vi "2048_game.vi"() -> ()   [LabVIEW 2021]
uses:
  gameover.ctl
  <vilib>/event_ctls.llb/eventvkey.ctl
panel:
  in  "module path 2":path
  in  "module path":path
  in  "AI":bool
  in  "player 2":bool
  in  "path 2":path
  in  "path":path
  in  "gameover 2":T1
  out "title 2":string
  out "summon_ani 2":u16[][](array[ring]) caption="Ring"
  in  "new game 2":bool
  out "P2 Score":i32
  out "Board 2":u16[][](array[ring])
  out "title":string
  in  "gameover":T1
  out "summon_ani":u16[][](array[ring]) caption="Ring"
  in  "new game":bool
  out "P1 Score":i32
  in  "stop":bool
  out "Board":u16[][](array[ring])
  # "P2控制方式\n上:W\n下:S\n左:A\n右:D"
  # "P1控制方式\n上:up\n下:down\n左:left\n右:right"
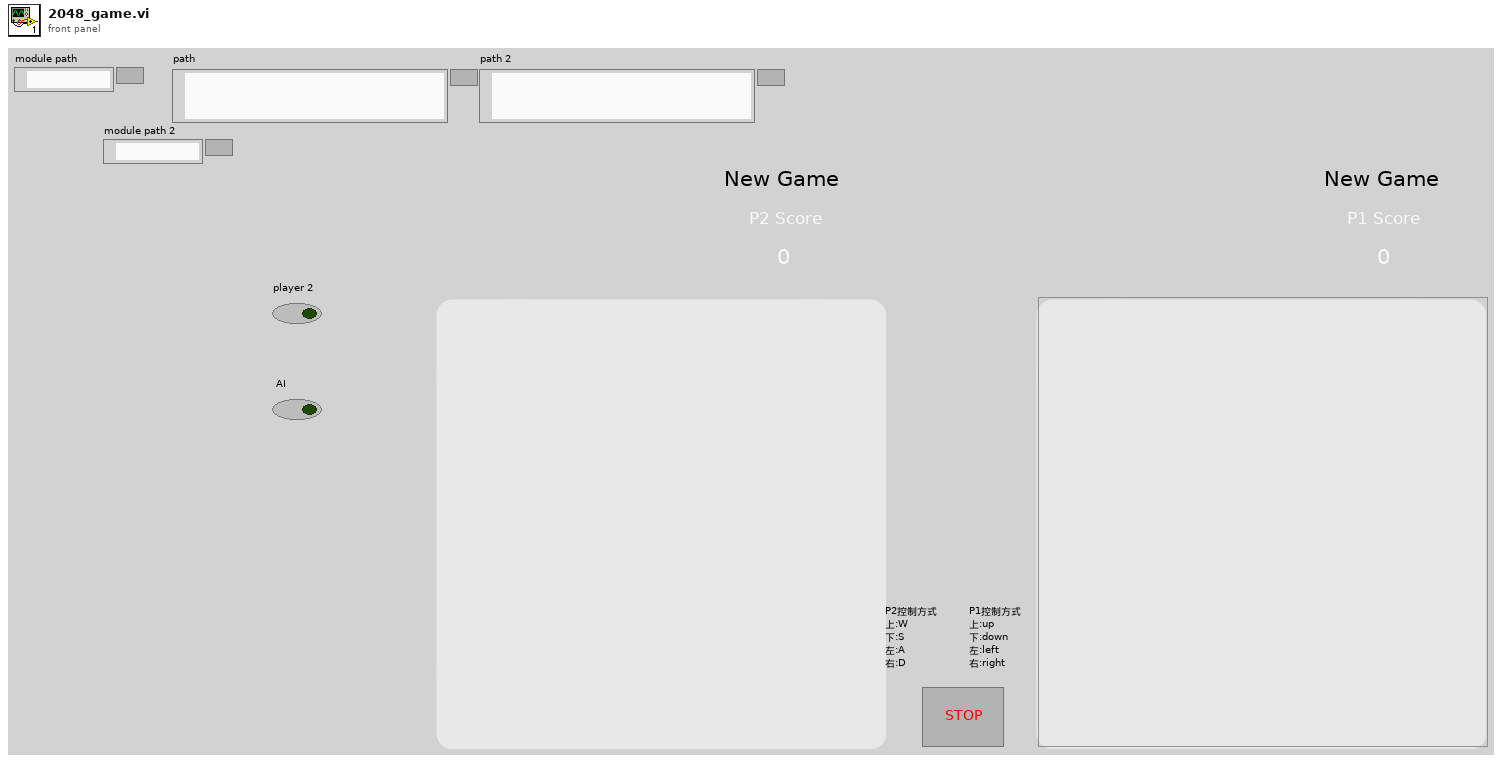
[diagram p1: front panel]
types:
  T1 = typedef "gameover.ctl" = bool
  T2 = typedef "Sound Output Task ID.ctl" = u32
  T3 = typedef "eventvkey.ctl" = enum16{"ASCII", "Enter", "Return", "Shift", "Ctrl", "Alt", "Cmd", "Opt", "Caps", "NumLock", "Clear", "Break", "Up", "Down", "Left", "Right", "Insert", "Delete", "Home", "End", "PageUp", "PageDown", "Escape", "Help", "Pause", "ScrollLock", "F1", "F2", "F3", "F4", "F5", "F6", "F7", "F8", "F9", "F10", "F11", "F12", "F13", "F14", "F15", "F16", "F17", "F18", "F19", "F20", "F21", "F22", "F23", "F24", "Play", "VolumeUp", "VolumeDown", "Mute", "Two Byte Char"}
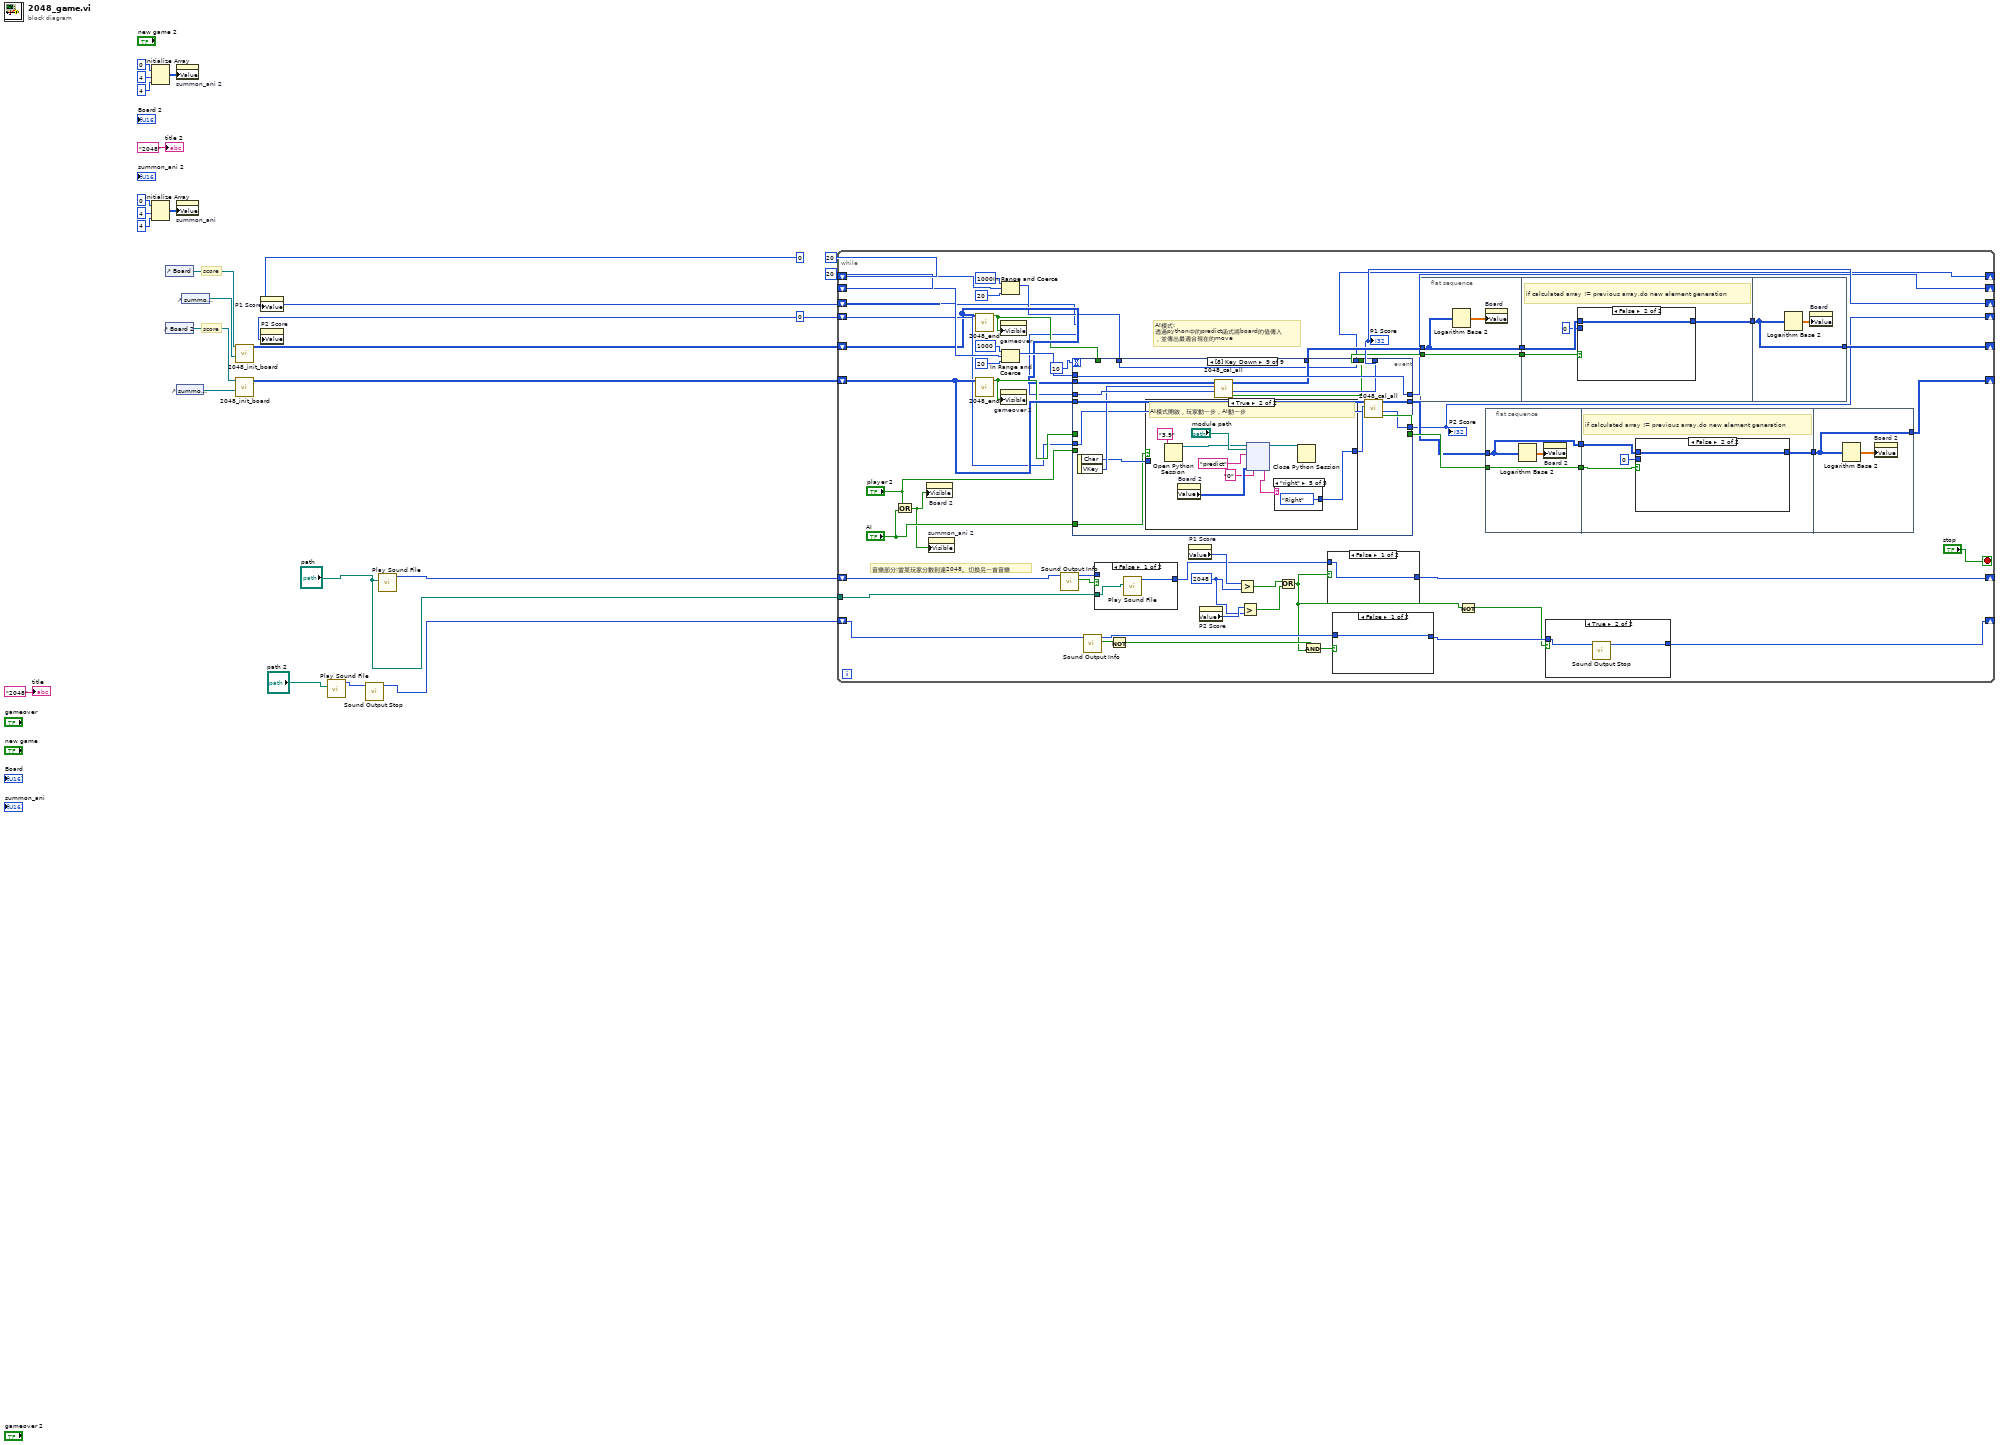
[diagram p0: block diagram]
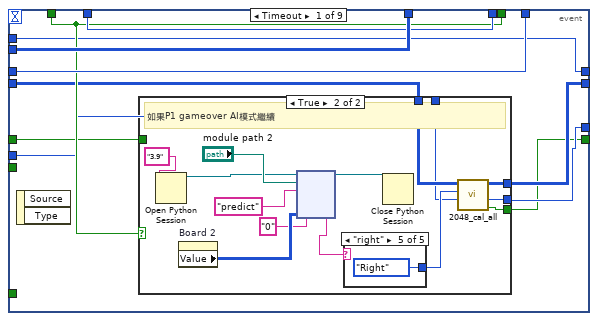
[diagram p2: hidden frame]
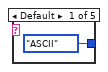
[diagram p4: hidden frame]
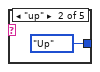
[diagram p5: hidden frame]
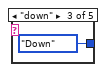
[diagram p6: hidden frame]
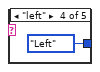
[diagram p7: hidden frame]
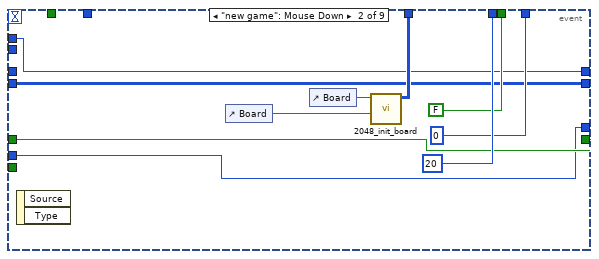
[diagram p8: hidden frame]
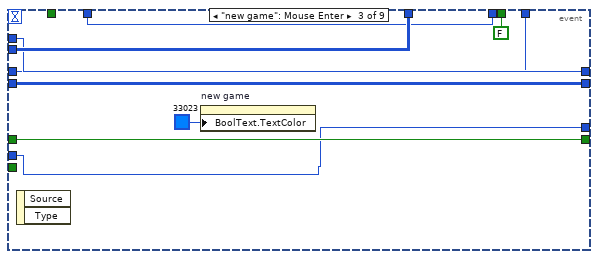
[diagram p9: hidden frame]
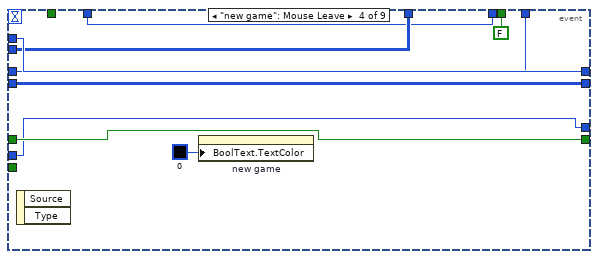
[diagram p10: hidden frame]
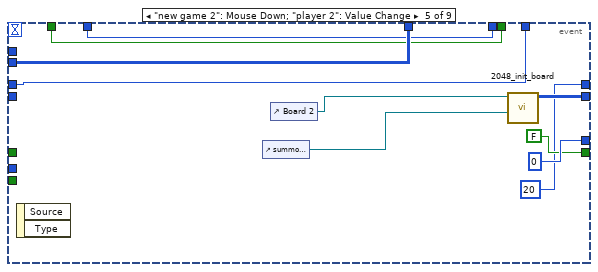
[diagram p11: hidden frame]
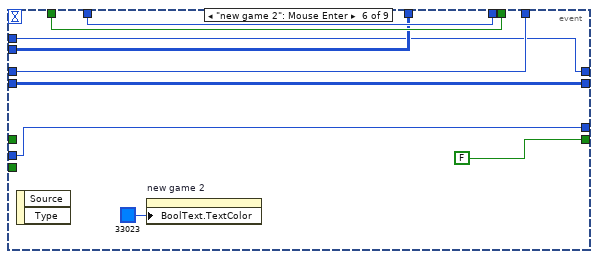
[diagram p12: hidden frame]
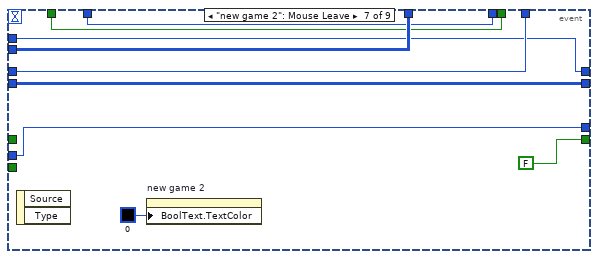
[diagram p13: hidden frame]
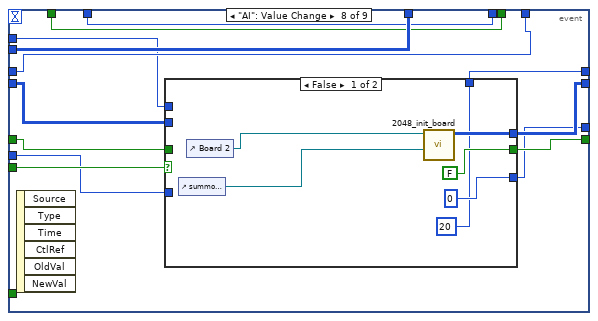
[diagram p14: hidden frame]
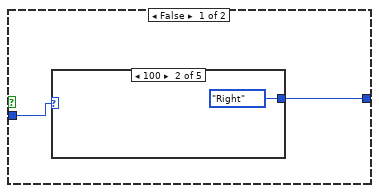
[diagram p16: hidden frame]
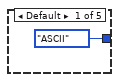
[diagram p17: hidden frame]
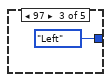
[diagram p18: hidden frame]
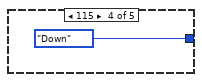
[diagram p19: hidden frame]
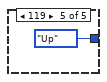
[diagram p20: hidden frame]
diagram:
  w9 = 0
  w12 = 0
  # "score"
  # "score"
  n1 = Initialize Array(0 ("element"), 4 ("dimension size"), 4 ("dimension size")) -> (w17:i32[][])
  n2 = Initialize Array(0 ("element"), 4 ("dimension size"), 4 ("dimension size")) -> (w25:i32[][])
  n3 = control-ref of="Board"() -> (w14:refnum<vi>)
  n4 = control-ref of="Board 2"() -> (w6:refnum<vi>)
  n5 = property on="summon_ani 2" class="Arr (strict)"("Value"=w17) -> ()  [unwired: 2 in, 2 out]
  n6 = property on="summon_ani" class="Arr (strict)"("Value"=w25) -> ()  [unwired: 2 in, 2 out]
  n7 = control-ref of="summon_ani 2"() -> (w7:refnum<vi>)
  n8 = control-ref of="summon_ani"() -> (w15:refnum<vi>)
  n9 = call "2048_init_board.vi"("summon_ani"=w15, "Array in"=w14) -> ("Array out"=w13:i32[][])  [unwired: 9 in]
  n10 = call "2048_init_board.vi"("summon_ani"=w7, "Array in"=w6) -> ("Array out"=w8:i32[][])  [unwired: 9 in]
  n11 = property on="P1 Score" class="DigNum (strict)"("Value"=w12) -> ()  [unwired: 2 in, 2 out]
  n12 = property on="P2 Score" class="DigNum (strict)"("Value"=w9) -> ()  [unwired: 2 in, 2 out]
  n13 = call <vilib>:"Play Sound File.vi"("path"="path 2") -> ("task ID"=w4:T2)  [unwired: 9 in, 1 out]
  n14 = call <vilib>:"Sound Output Stop.vi"("task ID"=w4) -> ("task ID out"=w3:T2)  [unwired: 9 in, 1 out]
  n15 = call <vilib>:"Play Sound File.vi"("path"="path") -> ("task ID"=w5:T2)  [unwired: 9 in, 1 out]
  n16 = while {
    shift-right: [w76] -> _
    shift-left: w13 -> [w37]
    shift-right: [w32] -> _
    shift-left: w12 -> [w34]
    shift-right: [w29] -> _
    shift-left: 20 -> [w73]
    shift-right: [w71] -> _
    shift-left: w8 -> [w44]
    shift-right: [w39] -> _
    shift-left: w9 -> [w42]
    shift-right: [w30] -> _
    shift-left: 20 -> [w72]
    shift-right: [w50] -> _
    shift-left: w5 -> [w52]
    shift-right: [w48] -> _
    shift-left: w3 -> [w51]
    tunnel: "path" -> [w53]
    stop <- "stop" stop-if-true
    w54 = 2048 ("y")
    # "AI模式: \n透過python中的predict函式將board的值傳入\n，並傳出最適合現在的move"
    # "音樂部分:當某玩家分數到達2048。切換另一首音樂"
    n17 = Or(x="player 2", y="AI") -> (x .or. y?=w27:bool)
    n18 = property on="Board 2" class="Arr (strict)"("Visible"=w27) -> ()  [unwired: 2 in, 2 out]
    n19 = property on="summon_ani 2" class="Arr (strict)"("Visible"=w27) -> ()  [unwired: 2 in, 2 out]
    n20 = call "2048_end.vi"("Array in"=w37) -> ("Boolean"=w36:bool)  [unwired: 10 in]
    n21 = call "2048_end.vi"("Array in"=w44) -> ("Boolean"=w43:bool)  [unwired: 10 in]
    n22 = property on="gameover" class="Bool (strict)"("Visible"=w36) -> ()  [unwired: 2 in, 2 out]
    n23 = property on="gameover 2" class="Bool (strict)"("Visible"=w43) -> ()  [unwired: 2 in, 2 out]
    n24 = In Range and Coerce(upper limit=1000, x=w73, lower limit=20) -> (coerced(x)=w35:i32)  [unwired: 1 out]
    n25 = In Range and Coerce(upper limit=1000, x=w72, lower limit=20) -> (coerced(x)=w38:i32)  [unwired: 1 out]
    n26 = call <vilib>:"Sound Output Info.vi"("task ID"=w52) -> ("is playing?"=w65:bool, "task ID out"=w64:T2)  [unwired: 7 in, 2 out]
    n27 = event shown="[8] Key Down" {
      selector: _ -> [_ _ _ _ _ _ _ _ _]
      dyn-events: _ -> [_ _ _ _ _ _ _ _ _]
      timeout: 10 -> [_ _ _ _ _ _ _ _ _]
      tunnel: [w86 w116 w129 w135 w151 w159 w168 w180 w206] -> w40
      tunnel: w44 -> [w87 w116 w129 w135 _ w159 w168 w175 w208]
      tunnel: [w82 w115 w130 w134 FALSE ("valid move") FALSE ("valid move") FALSE ("valid move") w178 w207] -> w41
      tunnel: [w84 w114 w124 w133 0 ("score") w153 w162 w176 w195] -> w39
      tunnel: w38 -> [w83 w117 w126 w139 _ w152 w161 w170 w205]
      tunnel: w43 -> [w81 w115 w130 w134 _ _ _ w174 _]
      tunnel: [w83 w117 w126 w139 20 w152 w161 w177 w205] -> w30
      tunnel: [w89 20 w127 w137 w146 w157 w165 w171 w197] -> w29
      tunnel: [w88 FALSE ("valid move") FALSE ("valid move") FALSE ("valid move") w144 w156 w164 w179 w198] -> w31
      tunnel: [w90 0 ("score") w125 w136 w145 w154 w163 w172 w199] -> w32
      tunnel: [w91 w118 w128 w138 w147 w155 w166 w181 w200] -> w33
      tunnel: w34 -> [w90 _ w125 w136 w145 w154 w163 w172 w203]
      tunnel: w37 -> [w91 _ w128 w138 w147 w155 w166 w181 w202]
      tunnel: w36 -> [w88 _ _ _ w144 w156 w164 w179 _]
      tunnel: w35 -> [w89 _ w127 w137 w146 w157 w165 w171 w197]
      tunnel: w42 -> [w85 w114 w124 w133 _ w153 w162 w173 w194]
      tunnel: "AI" -> [_ _ _ _ _ _ _ _ w193]
      tunnel: "player 2" -> [_ _ _ _ _ _ _ w182 _]
      event Timeout {
        n28 = event-data() -> ()  [unwired: 1 in, 2 out]
        n29 = case shown="True" w88 {
          tunnel: w87 -> [w94 w100]
          tunnel: [w94 w98] -> w86
          tunnel: w85 -> [w93 w97]
          tunnel: [w93 w96] -> w84
          tunnel: [w92 w95] -> w82
          tunnel: w81 -> [w92 _]
          frame False {
          }
          frame True {
            # "如果P1 gameover AI模式繼續"
            n30 = Open Python Session(python version="3.9" ("Python version")) -> (session out=w105:refnum<k35>)  [unwired: 2 in, 1 out]
            n31 = property on="Board 2" class="Arr (strict)"() -> ("Value"=w108:u16[][])  [unwired: 2 in, 2 out]
            n32 = node(w105, "module path 2", "predict" ("function name"), "0", w108) -> (w107:refnum<k35>, w104:string)  [unwired: 2 in, 3 out]
            n33 = case shown="\"right\"" w104 {
              tunnel: [eventvkey."ASCII" ("VKey in") eventvkey."Up" ("VKey in") eventvkey."Down" ("VKey in") eventvkey."Left" ("VKey in") eventvkey."Right" ("VKey in")] -> w99
              frame Default {
              }
              frame "up" {
              }
              frame "down" {
              }
              frame "left" {
              }
              frame "right" {
              }
            }
            n34 = Close Python Session(session in=w107) -> ()  [unwired: 1 in, 1 out]
            n35 = call "2048_cal_all.vi"("score in"=w97, "VKey in"=w99, "matrix"=w100) -> ("valid move"=w95:bool, "score out"=w96:i32, "matrix out"=w98:i32[][])  [unwired: 5 in, 1 out]
          }
        }
      }
      event "new game": Mouse Down {
        n36 = event-data() -> ()  [unwired: 1 in, 2 out]
        n37 = control-ref of="Board"() -> (w122:refnum<vi>)
        n38 = control-ref of="Board"() -> (w123:refnum<vi>)
        n39 = call "2048_init_board.vi"("summon_ani"=w122, "Array in"=w123) -> ("Array out"=w118:i32[][])  [unwired: 9 in]
      }
      event "new game": Mouse Enter {
        n40 = event-data() -> ()  [unwired: 1 in, 2 out]
        n41 = property on="new game" class="Bool (strict)"("BoolText.TextColor"=u32 33023 ("Boolean Text.Text Colors:Text Color")) -> ()  [unwired: 2 in, 2 out]
      }
      event "new game": Mouse Leave {
        n42 = event-data() -> ()  [unwired: 1 in, 2 out]
        n43 = property on="new game" class="Bool (strict)"("BoolText.TextColor"=u32 0 ("Boolean Text.Text Colors:Text Color")) -> ()  [unwired: 2 in, 2 out]
      }
      event "new game 2": Mouse Down; "player 2": Value Change {
        n44 = event-data() -> ()  [unwired: 1 in, 2 out]
        n45 = control-ref of="summon_ani 2"() -> (w143:refnum<vi>)
        n46 = control-ref of="Board 2"() -> (w142:refnum<vi>)
        n47 = call "2048_init_board.vi"("summon_ani"=w143, "Array in"=w142) -> ("Array out"=w151:i32[][])  [unwired: 9 in]
      }
      event "new game 2": Mouse Enter {
        n48 = event-data() -> ()  [unwired: 1 in, 2 out]
        n49 = property on="new game 2" class="Bool (strict)"("BoolText.TextColor"=u32 33023 ("Boolean Text.Text Colors:Text Color")) -> ()  [unwired: 2 in, 2 out]
      }
      event "new game 2": Mouse Leave {
        n50 = event-data() -> ()  [unwired: 1 in, 2 out]
        n51 = property on="new game 2" class="Bool (strict)"("BoolText.TextColor"=u32 0 ("Boolean Text.Text Colors:Text Color")) -> ()  [unwired: 2 in, 2 out]
      }
      event "AI": Value Change {
        n52 = event-data() -> ()  [unwired: 1 in, 6 out]
        n53 = case shown="False" w182 {
          tunnel: [w186 w192] -> w180
          tunnel: [0 ("score") w190] -> w176
          tunnel: [FALSE ("valid move") w191] -> w178
          tunnel: [20 w189] -> w177
          tunnel: w175 -> [_ w192]
          tunnel: w174 -> [_ w191]
          tunnel: w173 -> [_ w190]
          tunnel: w170 -> [_ w189]
          frame False {
            n54 = control-ref of="summon_ani 2"() -> (w188:refnum<vi>)
            n55 = control-ref of="Board 2"() -> (w187:refnum<vi>)
            n56 = call "2048_init_board.vi"("summon_ani"=w188, "Array in"=w187) -> ("Array out"=w186:i32[][])  [unwired: 9 in]
          }
          frame True {
          }
        }
      }
      event Key Down {
        n57 = event-data() -> ("Char"=w196:i16, "VKey"=w201:T3)  [unwired: 1 in]
        n58 = case shown="True" w193 {
          tunnel: [w210 w216] -> w204
          tunnel: w196 -> [w209 _]
          frame False {
            n59 = case shown="100" w209 {
              tunnel: [eventvkey."ASCII" ("VKey in") eventvkey."Right" ("VKey in") eventvkey."Left" ("VKey in") eventvkey."Down" ("VKey in") eventvkey."Up" ("VKey in")] -> w210
              frame Default {
              }
              frame 100 {
              }
              frame 97 {
              }
              frame 115 {
              }
              frame 119 {
              }
            }
          }
          frame True {
            # "AI模式開啟，玩家動一步，AI動一步"
            n60 = Open Python Session(python version="3.9" ("Python version")) -> (session out=w221:refnum<k35>)  [unwired: 2 in, 1 out]
            n61 = property on="Board 2" class="Arr (strict)"() -> ("Value"=w224:u16[][])  [unwired: 2 in, 2 out]
            n62 = node(w221, "module path", "predict" ("function name"), "0", w224) -> (w223:refnum<k35>, w217:string)  [unwired: 2 in, 3 out]
            n63 = case shown="\"right\"" w217 {
              tunnel: [eventvkey."ASCII" ("VKey in") eventvkey."Up" ("VKey in") eventvkey."Down" ("VKey in") eventvkey."Left" ("VKey in") eventvkey."Right" ("VKey in")] -> w216
              frame Default {
              }
              frame "up" {
              }
              frame "down" {
              }
              frame "left" {
              }
              frame "right" {
              }
            }
            n64 = Close Python Session(session in=w223) -> ()  [unwired: 1 in, 1 out]
          }
        }
        n65 = call "2048_cal_all.vi"("score in"=w203, "VKey in"=w201, "matrix"=w202) -> ("valid move"=w198:bool, "score out"=w199:i32, "matrix out"=w200:i32[][])  [unwired: 5 in, 1 out]
        n66 = call "2048_cal_all.vi"("score in"=w194, "VKey in"=w204, "matrix"=w208) -> ("valid move"=w207:bool, "score out"=w195:i32, "matrix out"=w206:i32[][])  [unwired: 5 in, 1 out]
      }
    }
    "P1 Score" <- w32
    "P2 Score" <- w39
    n67 = call <vilib>:"Sound Output Info.vi"("task ID"=w51) -> ("is playing?"=w58:bool, "task ID out"=w55:T2)  [unwired: 7 in, 2 out]
    n68 = case shown="False" w65 {
      tunnel: w64 -> [_ w241]
      tunnel: [w240 w241] -> w59
      tunnel: w53 -> [w239 _]
      frame False {
        n69 = call <vilib>:"Play Sound File.vi"("path"=w239) -> ("task ID"=w240:T2)  [unwired: 9 in, 1 out]
      }
      frame True {
      }
    }
    n70 = Not(x=w58) -> (.not. x?=w57:bool)
    n71 = property on="P1 Score" class="DigNum (strict)"() -> ("Value"=w63:i32)  [unwired: 2 in, 2 out]
    n72 = property on="P2 Score" class="DigNum (strict)"() -> ("Value"=w62:i32)  [unwired: 2 in, 2 out]
    n73 = Greater?(x=w63, y=w54) -> (0:w61:bool)
    n74 = Greater?(x=w62, y=w54) -> (0:w60:bool)
    n75 = Or(x=w61, y=w60) -> (x .or. y?=w47:bool)
    n76 = And(x=w57, y=w47) -> (x .and. y?=w56:bool)
    n77 = case shown="False" w47 {
      tunnel: w59 -> [w236 w238]
      tunnel: [w236 w237] -> w50
      frame False {
      }
      frame True {
        n78 = call <vilib>:"Sound Output Stop.vi"("task ID"=w238) -> ("task ID out"=w237:T2)  [unwired: 9 in, 1 out]
      }
    }
    n79 = case shown="False" w56 {
      tunnel: w55 -> [w233 w235]
      tunnel: [w233 w234] -> w49
      frame False {
      }
      frame True {
        n80 = call <vilib>:"Sound Output Start.vi"("task ID"=w235) -> ("task ID out"=w234:T2)  [unwired: 9 in, 1 out]
      }
    }
    n81 = flat-sequence {
      tunnel: w33 -> [w259]
      tunnel: w31 -> [w260]
      tunnel: [w260] -> w79
      tunnel: [w259] -> w78
      tunnel: w79 -> [w265]
      tunnel: w78 -> [w264]
      tunnel: [w263] -> w77
      tunnel: w77 -> [w274]
      tunnel: [w274] -> w76
      frame #0 {
        n82 = Logarithm Base 2(1:w259) -> (0:w261:dbl[][])
        n83 = property on="Board" class="Arr (strict)"("Value"=w261) -> ()  [unwired: 2 in, 2 out]
      }
      frame #1 {
        # "if calculated array != previous array,do new element generation"
        n84 = case shown="False" w265 {
          tunnel: w264 -> [w272 w273]
          tunnel: [w271 w273] -> w263
          tunnel: 0 -> [w270 _]
          frame True {
            n85 = control-ref of="summon_ani"() -> (w269:refnum<vi>)
            n86 = call "2048_generate_new_element.vi"("Array in"=w272) -> ("c"=w268:u64, "r"=w267:u64, "element"=w266:i16, "Array out"=w271:i32[][])  [unwired: 7 in]
            n87 = call "2048_summon_ani.vi"("speed"=w270, "Array in"=w269, "c"=w268, "r"=w267, "element"=w266) -> ()  [unwired: 7 in]
          }
          frame False {
          }
        }
      }
      frame #2 {
        n88 = Logarithm Base 2(1:w274) -> (0:w275:dbl[][])
        n89 = property on="Board" class="Arr (strict)"("Value"=w275) -> ()  [unwired: 2 in, 2 out]
      }
    }
    n90 = Not(x=w47) -> (.not. x?=w46:bool)
    n91 = flat-sequence {
      tunnel: w40 -> [w242]
      tunnel: w41 -> [w243]
      tunnel: [w243] -> w70
      tunnel: [w242] -> w69
      tunnel: w70 -> [w248]
      tunnel: w69 -> [w247]
      tunnel: [w246] -> w68
      tunnel: w68 -> [w257]
      tunnel: [w257] -> w71
      frame #0 {
        n92 = Logarithm Base 2(1:w242) -> (0:w244:dbl[][])
        n93 = property on="Board 2" class="Arr (strict)"("Value"=w244) -> ()  [unwired: 2 in, 2 out]
      }
      frame #1 {
        # "if calculated array != previous array,do new element generation"
        n94 = case shown="False" w248 {
          tunnel: w247 -> [w255 w256]
          tunnel: [w254 w256] -> w246
          tunnel: 0 -> [w253 _]
          frame True {
            n95 = control-ref of="summon_ani 2"() -> (w252:refnum<vi>)
            n96 = call "2048_generate_new_element.vi"("Array in"=w255) -> ("c"=w251:u64, "r"=w250:u64, "element"=w249:i16, "Array out"=w254:i32[][])  [unwired: 7 in]
            n97 = call "2048_summon_ani.vi"("speed"=w253, "Array in"=w252, "c"=w251, "r"=w250, "element"=w249) -> ()  [unwired: 7 in]
          }
          frame False {
          }
        }
      }
      frame #2 {
        n98 = Logarithm Base 2(1:w257) -> (0:w258:dbl[][])
        n99 = property on="Board 2" class="Arr (strict)"("Value"=w258) -> ()  [unwired: 2 in, 2 out]
      }
    }
    n100 = case shown="True" w46 {
      tunnel: w49 -> [w230 w232]
      tunnel: [w230 w231] -> w48
      frame False {
      }
      frame True {
        n101 = call <vilib>:"Sound Output Stop.vi"("task ID"=w232) -> ("task ID out"=w231:T2)  [unwired: 9 in, 1 out]
      }
    }
  }
  "title" <- "2048" ("title")
  "title 2" <- "2048" ("title 2")
